vi "CH375_Rel.vi"(8 "Error In":errorcluster caption="错误输入", 11 "移动步长":dbl) -> (0 "Error Out":errorcluster caption="错误输出")   [LabVIEW 2020]
uses:
  Global_CH375.vi
  <vilib>/Utility/config.llb/Write Key (String).vi
  lib/CH375/CH375.lvlib
  <vilib>/Utility/config.llb/NI_LVConfig.lvlib
panel:
  out "开始时间":dbl
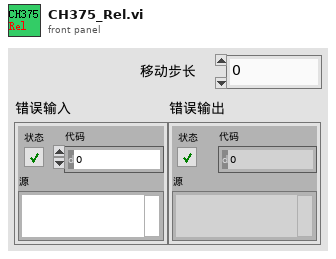
[diagram p1: front panel]
types:
  T1 = typedef "NI_LVConfig.lvlib/Config Data RefNum.ctl" = refnum<k1>
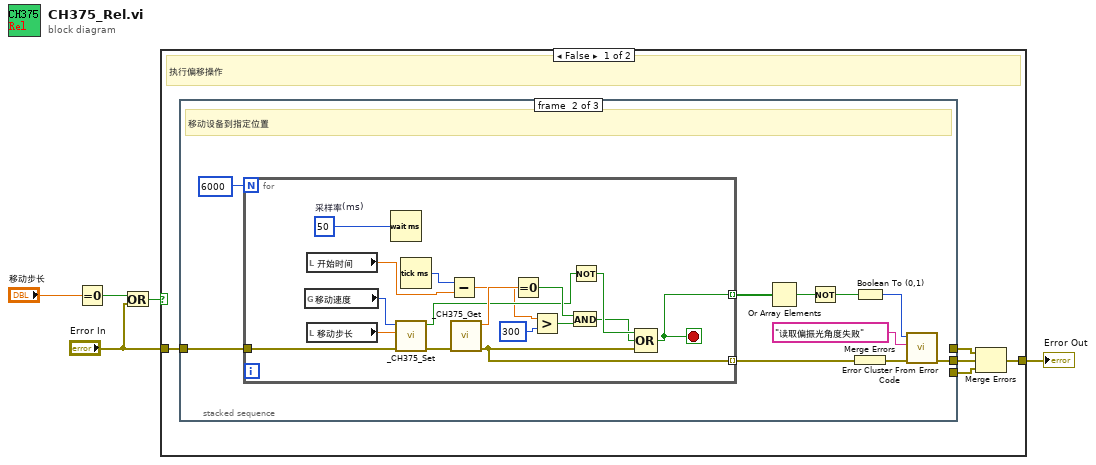
[diagram p0: block diagram]
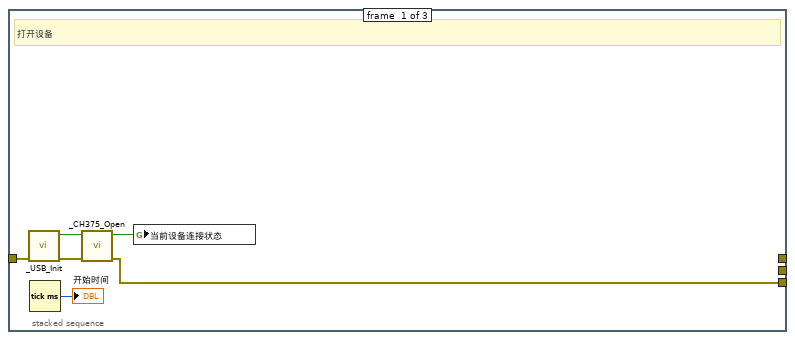
[diagram p2: hidden frame]
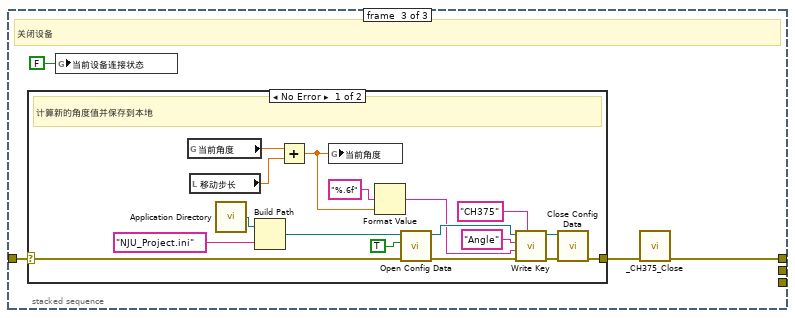
[diagram p3: hidden frame]
diagram:
  n1 = Equal To 0?(x="移动步长") -> (x = 0?=w3:bool)
  n2 = Or(x=w3, y="Error In") -> (x .or. y?=w2:bool)
  n3 = case shown="False" w2 {
    tunnel: [w10 w66] -> w5
    tunnel: "Error In" -> [w6 w66]
    frame False {
      # "执行偏移操作"
      n4 = stacked-sequence {
        tunnel: w6 -> [w13 w18 w45]
        tunnel: [w11 _ _] -> w8
        tunnel: [_ w17 _] -> w7
        tunnel: [_ _ w44] -> w9
        frame #0 {
          # "打开设备"
          n5 = call "_USB_Init.vi"("Error In"=w13) -> ("Error Out"=w16:errorcluster, "设备状态"=w15:bool)  [unwired: 9 in]
          n6 = Tick Count (ms)() -> (millisecond timer value=→"开始时间":u32)
          n7 = call "_CH375_Open.vi"("Error In"=w16, "USB状态"=w15) -> ("Error Out"=w11:errorcluster, "设备连接状况"=w12:bool)  [unwired: 8 in]
          n8 = global write "Global_CH375.vi" "当前设备连接状态"(w12) -> ()
        }
        frame #1 {
          # "移动设备到指定位置"
          n9 = for {
            N: 6000 -> [_]
            tunnel: [w30] -> w25 mode=indexing
            tunnel: [w28] -> w22 mode=indexing
            tunnel: w18 -> [w36]
            stop <- w28 stop-if-true
            w39 = 50  # 采样率(ms)
            n10 = global read "Global_CH375.vi" "移动速度"() -> (w38:u16)
            n11 = local read "开始时间"() -> (w33:dbl)
            n12 = local read "移动步长"() -> (w27:dbl)
            n13 = Wait (ms)(milliseconds to wait=w39) -> ()  [unwired: 1 out]
            n14 = call "_CH375_Set.vi"("Error In"=w36, "设定角度"=w27, "移动速度"=w38) -> ("Error Out"=w37:errorcluster, "设置成功"=w35:bool)  [unwired: 7 in]
            n15 = Tick Count (ms)() -> (millisecond timer value=w32:u32)
            n16 = Subtract(x=w32, y=w33) -> (x-y=w31:dbl)
            n17 = call "_CH375_Get.vi"("Error In"=w37) -> ("Error Out"=w30:errorcluster, "实时角度(参考值)"=w43:dbl)  [unwired: 9 in]
            n18 = Equal To 0?(x=w43) -> (x = 0?=w41:bool)
            n19 = Greater?(x=w31, y=300) -> (0:w40:bool)
            n20 = And(x=w41, y=w40) -> (x .and. y?=w29:bool)
            n21 = Not(x=w35) -> (.not. x?=w34:bool)
            n22 = Compound Arithmetic op=OR(w34, w29, w30) -> (w28:bool)
          }
          n23 = Or Array Elements(Boolean array=w22) -> (logical OR=w20:bool)
          n24 = Not(x=w20) -> (.not. x?=w19:bool)
          n25 = Boolean To (0,1)(Boolean=w19) -> (0, 1=w21:i16)
          n26 = Merge Errors(w25) -> (w26:errorcluster)
          n27 = call <vilib>:"Error Cluster From Error Code.vi"("error in (no error)"=w26, "error message (\"\")"="读取偏振光角度失败", "error code (0)"=w21) -> ("error out"=w17:errorcluster)  [unwired: 6 in]
        }
        frame #2 {
          # "关闭设备"
          n28 = case shown="No Error" w45 {
            selector: w45 -> [w63 w65]
            tunnel: [w64 w65] -> w46
            frame No Error {
              # "计算新的角度值并保存到本地"
              n29 = global read "Global_CH375.vi" "当前角度"() -> (w51:dbl)
              n30 = local read "移动步长"() -> (w50:dbl)
              n31 = call <vilib>:"Application Directory.vi"() -> ("Application Directory"=w62:path)
              n32 = Build Path(base path=w62, name or relative path="NJU_Project.ini") -> (appended path=w61:path)
              n33 = Add(x=w51, y=w50) -> (x+y=w49:dbl)
              n34 = global write "Global_CH375.vi" "当前角度"(w49) -> ()
              n35 = Format Value(format string="%.6f", value (0)=w49) -> (output string=w54:string)  [unwired: 1 in]
              n36 = call <vilib>:"Open Config Data.vi"("error in (no error)"=w63, "create file if necessary (T)"=TRUE, "configuration file path"=w61) -> ("error out"=w59:errorcluster, "refnum"=w58:T1)  [unwired: 6 in, 1 out]
              n37 = call-poly <vilib>:"Write Key.vi"("section"="CH375", "error in (no error)"=w59, "value"=w54, "key"="Angle", "refnum"=w58) -> ("error out"=w53:errorcluster, "refnum out"=w52:T1)  [unwired: 4 in, 1 out]
              n38 = call <vilib>:"Close Config Data.vi"("error in (no error)"=w53, "refnum"=w52) -> ("error out"=w64:errorcluster)  [unwired: 8 in, 1 out]
            }
            frame Error {
            }
          }
          n39 = global write "Global_CH375.vi" "当前设备连接状态"(FALSE) -> ()
          n40 = call "_CH375_Close.vi"("Error In"=w46) -> ("Error Out"=w44:errorcluster)  [unwired: 10 in]
        }
      }
      n41 = Merge Errors(w9, w7, w8) -> (w10:errorcluster)
    }
    frame True {
      # "上一级发生错误活移动步长为0时"
    }
  }
  "Error Out" <- w5
